vi "ReceiveCRC.vi"(2 "error in":errorcluster caption="错误输入（无错误）", 3 "128K？":bool, 4 "StrIn":string) -> (0 "error out":errorcluster caption="错误输出", 1 "CRCStr":string)   [LabVIEW 2013]
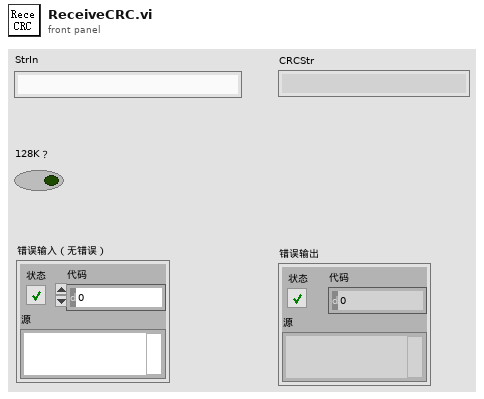
[diagram p1: front panel]
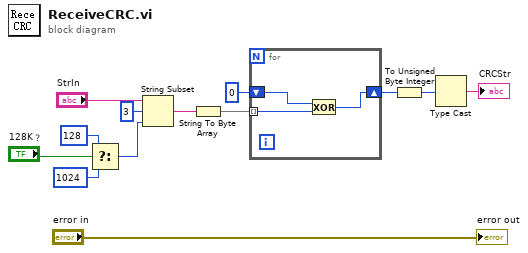
[diagram p0: block diagram]
diagram:
  n1 = Select(t=128 ("偏移量(0)"), s="128K？", f=1024 ("偏移量(0)")) -> (s? t:f=w2:i32)
  n2 = String Subset(string="StrIn", offset (0)=3 ("偏移量(0)"), length (rest)=w2) -> (substring=w10:string)
  n3 = String To Byte Array(string=w10) -> (unsigned byte array=w9:u8[])
  n4 = for {
    shift-right: [w14] -> w8
    shift-left: u8 0 -> [w16]
    tunnel: w9 -> [w15] mode=indexing
    n5 = Exclusive Or(1:w15, 2:w16) -> (0:w14:u8)
  }
  n6 = To Unsigned Byte Integer(number=w8) -> (unsigned 8bit integer=w7:u8)
  n7 = Type Cast(x=w7) -> (*(type *) &x=→"CRCStr":string)  [unwired: 1 in]
  "error out" <- "error in"
